vi "MainPanel_20170525.vi"() -> (0 "ErrorOut":errorcluster={"status"=TRUE, "code"=-63195, "source"="niLvFpga_Close_Dynamic.vi"})   [LabVIEW 2018]
doc: "This is the main application VI and is a good framework to begin all applications with. See block diagram for detailed documentation.\n\n\nCopyright © 2017 Epimedia, Inc. All Rights Reserved.\n\nThe Epimedia Application Library is Copyright © 2009-2017 Epimedia, Inc. \nAll Rights Reserved. Used under license."
uses:
  Controls/Clusts/FreqShift.ctl
  Controls/Enums/TargetNumber.ctl
  Controls/Clusts/ScaleTargetClust.ctl
  Controls/Clusts/FPGA_Scale.ctl
  Controls/RadioButtons/FilterEnableRadio.ctl
  Controls/Clusts/Inclinometer_User_Cfg.ctl
  Controls/Clusts/AlarmSettingsClust.ctl
  Controls/Clusts/AlarmThresh_OneChan.ctl
  Controls/Clusts/SaturationMonitor.ctl
  Queue/MainQueueElements.ctl
  Queue/HWQueueElements.ctl
  Queue/DataQueueElements.ctl
  Controls/MasterCluster.ctl
  Controls/Clusts/AdminCluster.ctl
  Controls/UserLevelEnum.ctl
  Controls/RT_Config.ctl
  Controls/SMSDataCluster.ctl
  Controls/Clusts/FPGA_Config_Clust.ctl
  Controls/Clusts/Config_Clust.ctl
  Controls/Clusts/UserConfig.ctl
  Controls/PathsCluster.ctl
  Controls/Clusts/FrontPanel_UserConfig.ctl
  Controls/Clusts/FP_UserTargetConfig.ctl
  Controls/Enums/ScaleMeasure.ctl
  Controls/SystemStatusCluster.ctl
  Controls/SystemStateEnum.ctl
  Controls/Enums/NoiseQueueElements.ctl
  Controls/Enums/DigiLoopEnum.ctl
  Controls/Enums/FP_Loop_Enum.ctl
  Controls/Enums/AI_Type_Enum.ctl
  Controls/Clusts/FP_Loop_Clust.ctl
  Controls/Clusts/DigOutClust.ctl
  Controls/Clusts/NoiseFLoorSums.ctl
  Controls/Clusts/PowerHistory_All.ctl
  Controls/Enums/10Hz_Loop_Enum.ctl
  Controls/Enums/TCP_Loop.ctl
  Controls/Enums/LogLoopEnum.ctl
  Controls/Clusts/HDF5_10HzRefs.ctl
  <vilib>/addons/h5labview2/base/hid_t.ctl
  Controls/Clusts/TargetToneData.ctl
  Controls/Clusts/ChannelToneData.ctl
  Controls/ToneInfoClust.ctl
  Controls/Enums/WatchdogTimer_Enum.ctl
  Controls/Clusts/NoiseFloorData.ctl
  Controls/Clusts/FPGA_Probes.ctl
  Controls/Clusts/PXI_Health.ctl
  Controls/Clusts/All_AI_Error_and_Data.ctl
  Controls/Clusts/AI_Clust.ctl
  Controls/Clusts/All_AI_Error_Status.ctl
  Controls/Clusts/ErrorStatus.ctl
  Controls/Clusts/All_TC_Error_and_Data.ctl
  HDF5/TC_Data_Structure.ctl
  Controls/Clusts/All_TC_Error_Status.ctl
  Controls/Clusts/AlarmDisplay.ctl
  Controls/Clusts/SerialMeasurements_Clust.ctl
  Controls/Clusts/Saturation_Status_Clust.ctl
  Controls/Enums/AI_Loop_Enum.ctl
  Controls/Enums/AO_Loop_Enum.ctl
  <vilib>/Utility/xml.llb/Write to XML File(string).vi
panel:
  out "TCP Connection":bool=TRUE
  out "Cx_Yell":bool
  out "Red":bool
  out "Rx_Yell":bool
  out "Green":bool=TRUE
  out "Logging to NAS":bool=TRUE
  out "10 MHzPLL Status":bool
  out "Input Over Range":bool=TRUE
  out "Auto Center":bool
  in  "Location":string caption="Connex Location"
  out "UTC date/time":string
  in  "Config":bool
  in  "SysErr":string="\nUnrecoverable System Error Handling Error!\n\nKey System File(s) are missing.\n"
  in  "RightSideTab":T1(tab)
  in  "AutoOffset":bool caption="Auto Offset"
  out "84 GHz":T2 {"MeasMax" format="%#.2g"; "MeasMean1" format="%#.2g"; "7_Max" format="%#.6g"; "6_Max" format="%#.2g"; "5_Max" format="%#.2g"; "4_Max" format="%#.2g"; "1_Max" format="%#.2g"; "MeasMean0" format="%#.2g"}
  in  "Scale":T3={"Measure"=0.050018310546875, "Step1"=2.0, "Scale"={"Step4"=3.0, "Step5"=1.0, "Step6"=1.0, "Step7"=1.0}} caption="Scale All Targets" {"Step1" format="%#_4g"; "Measure" format="%#_4g"}
  in  "FilterEnable":T5=enum."Step 1" caption="Enable Filter Stages"
  out "72 GHz":T2 {"MeasMax" format="%#.2g"; "MeasMean1" format="%#.2g"; "7_Max" format="%#.6g"; "6_Max" format="%#.2g"; "5_Max" format="%#.2g"; "4_Max" format="%#.2g"; "1_Max" format="%#.2g"; "MeasMean0" format="%#.2g"}
  out "Digitizer Offset 72 Co":fxp<+/-,16,16> caption="72 Co"
  out "Digitizer Offset 72 X":fxp<+/-,16,16> caption="72 X"
  out "Digitizer Offset 84 Co":fxp<+/-,16,16> caption="84 Co"
  out "Digitizer Offset 84 x":fxp<+/-,16,16> caption="84 x"
  in  "SimulateFPGA":bool caption="Simulate FPGA Signal"
  out "Voltages":string[][](table)=[["5V Aux", "4.50", "5.50", "4.99", "Yes"], ["3.3V Aux", "2.97", "3.63", "3.25", "Yes"], ["5V Backplane", "4.50", "5.50", "4.98", "Yes"], ["3.3V Backplane", "2.97", "3.63", "3.29", "Yes"], ["12V Backplane", "10.80", "13.20", "11.95", "Yes"], ["-12V Backplane", "-13.20", "-10.80", "-11.86", "Yes"], ["12V Fan", "10.80", "13.20", "12.01", "Yes"]]
  out "Fans":string[][](table)=[["Fan 1", "2438"], ["Fan 2", "2438"], ["Fan 3", "2443"], ["Fan 4", "2437"], ["Fan 5", "2436"], ["Fan 6", "2440"]]
  out "Temperatures":string[][](table)=[["Intake", "-20.00", "200.00", "32.00", "Yes"], ["Exhaust Temp1", "-40.00", "85.00", "51.23", "Yes"], ["Exhaust Temp2", "-40.00", "85.00", "40.30", "Yes"], ["Exhaust Temp3", "-40.00", "85.00", "37.18", "Yes"], ["Exhaust Temp4", "-40.00", "85.00", "40.30", "Yes"]]
  out "Combined Power History":T6(graph)
  in  "NewValueWeighting":dbl=0.75 min=0.01 max=1.0 step=0.01
  in  "Inclin":T7
  out "Inclinometer History":T8(graph)
  in  "LeftSideTab":T9(tab)
  in  "Deadband":dbl caption="Tracking Deadband (Hz)\nfull width" format="%#.0f"
  in  "MaxTrackRate":u32 caption="Track Rate (df/s)"
  in  "SNR_Thresh":dbl=-90.0 caption="Don't AutoCenter below this SNR level (dB)"
  in  "Tone Tabs":T10(tab)
  out "Cal":dbl[](graph)
  out "Beacon":dbl[][](graph)
  out "FreqShiftTab_72Co":enum32{"Auto", "Manual"}(tab)=enum."Manual"
  in  "Shift Cal":T11={"Fine"=-2000.0, "Coarse_"=25000000.0} {"Coarse_" format="%_9f"; "Fine" step=100.0 format="%^#_6g"}
  in  "Shift Beac":T11={"Fine"=0.0, "Coarse_"=25624000.0} {"Coarse_" format="%_9f"; "Fine" step=500.0 format="%^#_6g"}
  out "Channel Power Cal":dbl
  out "Channel Power Beac":dbl
  out "Peak Location Cal":dbl format="%^#_9g"
  out "Peak Location Beacon":dbl format="%^#_9g"
  out "SNR":dbl
  out "Beacon 2":dbl[](graph)
  out "Cal 2":dbl[](graph)
  out "Channel Power Beac 2":dbl
  out "Channel Power Cal 2":dbl
  out "Peak Location Cal 2":dbl format="%^#_9g"
  out "Peak Location Beacon 2":dbl format="%^#_9g"
  out "SNR 2":dbl
  out "Peak Location Cal 3":dbl format="%^#_9g"
  out "Peak Location Beacon 3":dbl format="%^#_9g"
  out "Channel Power Beac 3":dbl
  out "Channel Power Cal 3":dbl
  out "Cal 3":dbl[](graph)
  out "Beacon 3":dbl[][](graph)
  out "FreqShiftTab_84Co":enum32{"Auto", "Manual"}(tab)=enum."Manual"
  in  "Shift Cal 3":T11={"Fine"=-2000.0, "Coarse_"=25000000.0} {"Coarse_" format="%_9f"; "Fine" step=1000.0 format="%^#_6g"}
  in  "Shift Beac 3":T11={"Fine"=-1200.0, "Coarse_"=25508000.0} {"Coarse_" format="%_9f"; "Fine" step=3000.0 format="%^#_6g"}
  out "SNR 3":dbl
  out "Peak Location Cal 4":dbl=25000867.0 format="%^#_9g"
  out "Peak Location Beacon 4":dbl=26247708.0 format="%^#_9g"
  out "Channel Power Beac 4":dbl=-172.30831588057904
  out "Channel Power Cal 4":dbl=-172.65485177884602
  out "Cal 4":dbl[](graph)
  out "Beacon 4":dbl[](graph)
  out "SNR 4":dbl
  out "df (Hz)":dbl=1.0
  in  "Zoom On Peak":bool
  in  "AutoCenter":bool
  in  "AutoScale Y Tones":bool caption="AutoScale Y"
  out "Delta Phase 84 GHz":dbl(graph)
  out "Delta Phase 72 GHz":dbl(graph)
  out "84 X Beac":dbl(graph)
  out "84 Co Beac":dbl(graph)
  out "72 X Beac":dbl(graph)
  out "72 Co Beac":dbl(graph)
  in  "NoiseCalcTabs":enum32{"Sums", "Calculations"}(tab)
  out "Noise Floor Sum Histories":cluster{"1":dbl, "2":dbl, "3":dbl, "4":dbl}(graph)
  out "NoiseFloorSum 2":dbl=7.853169888502882e-06 caption="NoiseFloorSum 72 X" format="%^#.4g"
  out "NoiseFloorSum 4":dbl caption="NoiseFloorSum 84 X" format="%^#.4g"
  out "NoiseFloorSum 3":dbl=5.6412082576295616e-06 caption="NoiseFloorSum 84 Co" format="%^#.4g"
  out "NoiseFloorSum":dbl=1.7031731794048579e-06 caption="NoiseFloorSum 72 Co" format="%^#.4g"
  in  "FreqsToRemove 2":i32[](array[numeric])=[0, 1633] caption="Frequencies to remove [Hz]" format="%#.9f"
  in  "Width 2 [bins]":i32[](array[numeric])
  in  "FreqsToRemove":i32[](array[numeric])=[0, 1633] caption="Frequencies to remove [Hz]" format="%#.9f"
  in  "Width [bins]":i32[](array[numeric])
  in  "Noise Floor Tabs":T10(tab)=enum."84 GHz Cross"
  out "NoiseFloor":dbl[](graph)=[-66.50915074981145, -77.35517980815544, -70.92434771683105, -72.86535876954508, -107.5864217084241, -66.94671114313334, -86.9680791592285, -68.04380719104392, -71.14797089641604, -63.16968529661337, -82.48880594923583, -62.394262379750494, -69.41405540583582, -70.44999041078472, -62.764694502724275, -69.85852362169294, -61.20801118479691, -60.96232819890859, -67.0420916611973, -76.9325123260613, -71.20470080745599, -59.94612909219138, -67.09384592930908, -67.75357665166754, -63.68561668587035, -79.05247609152548, -64.30819977245869, -71.92525230951662, -62.60086763754057, -76.64734907877724, -67.28855831253992, -67.13098496137215, -59.47573928376156, -63.37374642804294, -58.85306181225433, -59.0113657345912, -64.58953958406045, -70.86924704839845, -79.26102778332853, -61.52216258278157, -80.3481898614786, -75.765935107876, -65.48046717202362, -69.19931261895289, -63.949032467233216, -63.75864694613728, -72.87889864476392, -56.79760525136199, -71.65909904633395, -59.06578970836555, -64.91475716928525, -57.19343570542245, -62.79306219219861, -55.81556426495866, -64.05645800193233, -65.73443303002963, -75.21456372039822, -86.01638976497799, -53.953967724982654, -62.330882253021905, -62.661391497611554, -55.735821494891475, -77.26914335701082, -83.54061295051198, -55.53376160252768, -59.37242649088039, -60.48906914982559, -75.0602494009469, -66.65904341140876, -77.75218818680568, -52.477623238047464, -66.00191924743532, -81.95073969565235, -55.208321856836896, -81.91591933074315, -73.83258325532779, -60.85727300175419, -75.67483280875109, -105.75362882215944, -63.135275318647835, -86.90940619345022, -56.06589110459543, -62.14321627753413, -65.89664521425757, -71.08033489355404, -88.42724907547671, -86.34160735020279, -68.07660380418503, -74.5954456871255, -60.31196258100402, -102.29042779841981, -58.54712285471978, -57.1066682233888, -63.68561668587035, -53.84157042278512, -64.07808822530168, -83.09809005033009, -67.86540306368099, -59.74416373775657, -57.42602087556475, -82.86505025051522, -83.4178863299571, -61.36992220129098, -63.283623635764734, -62.448923496303216, -64.15963873058894, -79.77530324298593, -76.62730100460487, -58.90659256005497, -57.12238586753852, -64.13237812685045, -70.84729509373918, -62.27688773899296, -66.60253072956394, -67.06423788111388, -57.29166293696944, -62.40335096403998, -81.985686910987, -80.43715185916025, -64.04566115217133, -92.88133277427832, -55.42331829191223, -55.120674896161084, -63.194339640689996, -61.59292923045107, -60.29735024002179, -53.54632146630568, -81.64181496888733, -61.82980546303049, -57.78161308733092, -73.11204950616451, -60.511439156076044, -60.66950707129386, -57.55954298568111, -72.55910236513691, -67.66661849545392, -73.15378851327321, -80.11491392918538, -76.8092600952713, -57.76758207707761, -59.68576391549755, -69.68214071607247, -58.27721758621551, -57.474854125813316, -57.792852690256986, -71.61149100817491, -57.59528138494674, -64.40853421412848, -59.10117046934344, -62.085865451395556, -64.29711600461678, -70.94647690772834, -59.96021573202071, -71.40013117318102, -91.0059778265747, -68.6782163581475, -85.80554611282477, -64.97400998274259, -62.950601935766436, -55.110040819027354, -59.39233587194578, -76.10125856709311, -70.38708526734541, -63.70121929164116, -61.167956846856164, -56.64922452409264, -63.135275318647835, -73.04288554397968, -75.91352263430315, -58.88136440613294, -95.07660997858827, -76.9325123260613, -55.1933009388814, -65.66391951508285, -53.42073336253301, -61.02513038720361, -79.20846326824847, -59.627717466812165, -78.74791082859372, -79.00103897097017, -56.92260555741537, -53.90697537079881, -122.53370302934468, -60.593911723440904, -59.84809758215223, -55.827010394463606, -70.85826479190422, -63.071696702033954, -67.59605258674068, -59.827220533651264, -76.40949391870066, -61.136033356497144, -93.32759928426387, -60.677099473747965, -64.04026728078941, -59.69261605864603, -66.99795201277061, -65.4491890223706, -81.985686910987, -62.33991095957074, -69.97794010149332, -66.42113041531445, -64.87938036213663, -60.47790367814803, -58.27721758621551, -61.95047372074091, -67.30370117282712, -55.47838100766122, -82.34234508908514, -64.4253591234399, -62.10347536914477, -64.12149553918309, -70.89124935162172, -64.06726701716042, -65.83143082306387, -71.28469055024624, -65.3374246513794, -83.54061295051198, -70.71662792027197, -79.02672305592466, -71.5169779283971, -66.49745848526379, -61.685291431907324, -90.91673997376512, -61.46839697534468, -55.97939338197404, -71.99913970945016, -70.59839337034478, -58.73757611624553, -69.25487068930309, -71.44669922579382, -86.62130646331073, -56.72690106185417, -64.79733832268226, -71.3307002307699, -80.55706592055753, -68.08482050704285, -61.989584533692884, -59.67891666324396, -68.02745083584529, -57.598036015259986, -76.85016847282978, -62.14321627753413, -88.29117587199889, -53.237129671891786, -53.739683783843354, -69.11657420476445, -63.92236300329483, -57.9116704876057, -85.85782417136002, -60.08079476870609, -63.434302126231735, -82.78861159907069, -67.65089226242378, -67.23574575288268, -54.48667245338559, -67.36451278692888, -60.70752931686879, -69.02547190563956, -61.79133938342206, -74.10582008083972, -62.34442850144843, -53.97471751185552, -51.333739549665786, -65.72800124970155, -85.10207921011511, -67.70604723982245, -81.91591933074315, -57.87190081264216, -72.98791118149637, -65.14189176731313, -63.11077211247754, -61.02513038720361, -77.3768100315248, -69.61441375800541, -57.31303415160058, -78.21347897550834, -59.99198650623064, -59.114068622547016, -62.61480082808004, -65.28816652004411, -67.22070969964764, -73.65465543441897, -71.34223721351944, -67.02735586720914, -73.65465543441897, -56.18403299187383, -57.523937234598, -67.25834411433442, -77.05736875236039, -62.398805595558834, -59.63452825872057, -69.50894243068942, -55.60288055349337, -80.20172900132795, -79.44730548095569, -55.63875065838558, -66.10836139358406, -58.72207603208485, -58.29497692482666, -59.08185569771779, -72.67778016739874, -65.52442862375423, -61.98087945142586, -58.25949106438673, -59.88998847841493, -60.749528587935266, -84.40154908991724, -66.44881586021592, -53.29676818907982, -52.73633391630178, -60.71896543982064, -53.09135769185345, -58.6265305032935, -73.75804519578128, -56.71935642914125, -68.61719752452004, -57.598036015259986, -53.3337898283395, -64.87349689062438, -88.29117587199889, -58.453295635683695, -57.28632756419565, -61.12011136114078, -78.28462639681322, -66.36599807965678, -76.64734907877724, -59.63452825872057, -66.75159255224662, -65.43670626198858, -64.71599198424335, -90.23123413228441, -71.70694453204936, -61.660013419915934, -74.24541348985224, -75.82101468502773, -55.70410906931722, -64.08350341031704, -68.94421306683006, -57.3264153784878, -68.89936492530401, -77.18387168443718, -60.79171254557675, -58.58369087867003, -67.73770733456635, -65.3497788063386, -62.12995100692533, -61.02119318214117, -66.23631485249587, -53.28621676730112, -69.5759262439922, -69.46138159950439, -62.394262379750494, -89.51441115362678, -59.01455861197133, -66.53934938152648, -59.398981525138474, -61.28457827894233, -63.179539432045864, -71.50522899857577, -53.402925672251335, -72.18638703360062, -65.8184409768001, -77.26914335701082, -77.618018167542, -74.4029375547791, -65.92285561307659, -59.696043966490244, -89.74745095344164, -59.57340451210353, -54.16158766254612, -66.37975148703052, -59.09794863891852, -70.30384830260698, -58.90659256005497, -60.522643751470916, -76.68757135992576, -63.298585427204195, -69.00735480865882, -67.54152462831524, -59.823745438521804, -59.2636574163325, -68.09304425379594, -65.96230597710542, -74.5630915249219, -62.03760420165235, -59.188571445108, -59.96021573202071, -62.23212330872112, -67.46416130580153, -75.72939030177491, -62.77414108152802, -66.8957425222851, -68.37693094025309, -100.44500423225278, -67.67449129031516, -49.330032478862485, -65.90974146202535, -63.84279660853401, -78.3084599494455, -88.84744763463866, -70.68423734363549, -71.03550770917977, -66.0350557225249, -61.77003579927264, -66.27027241007812, -53.80810643536217, -73.95306207593867, -86.73551019305384, -58.65109645781953, -75.16284930944386, -66.04169677505735, -68.53069558583377, -91.655027241384, -65.83143082306387, -73.09817676332747, -87.63833899908943, -57.84642138199265, -71.35378808788312, -68.462051285777, -66.56036362870307, -69.74057541452339, -64.89115814139384, -72.19900110510912, -89.82640613165822, -74.43475516272025, -74.35540814293401, -57.55131453628453, -55.07397287871715, -62.462637580125666, -65.03363105719274, -73.07049131842601, -56.80014006442999, -57.398998322484964, -64.85586809546422, -56.72690106185417, -63.92236300329483, -72.71766795875487, -69.27346178039309, -60.188461443220056, -61.325123563306455, -66.22953774165236, -56.500646437883866, -80.1437650787519, -61.8469511333678, -64.06726701716042, -67.21320050161253, -75.02629184336465, -69.9180460463688, -64.76239110734761, -63.949032467233216, -59.18206991995233, -69.8981641739671, -60.7380559933847, -75.63863276579386, -103.86658696945702, -75.58458755242262, -70.34537650598938, -67.16826833515842, -64.37497266386126, -59.97785317034083, -87.38915615802296, -80.77059142903238, -98.69599353792836, -58.90659256005497, -68.81916287895487, -62.085865451395556, -67.92989406287103, -59.526131625169576, -80.0574706437699, -135.8324248355678, -65.53702613048907, -88.29117587199889, -75.33632600787547, -60.239122443647425, -57.73678590295665, -69.06180907029892, -58.72517404599841, -65.9031911032867, -69.4994113817186, -66.88848334675899, -66.8957425222851, -80.67849792174991, -69.67243611231109, -67.92180893807722, -70.89124935162172, -56.272404337593876, -66.0350557225249, -67.48730486346835, -60.533861449104684, -71.40013117318102, -87.45084768896143, -62.93617275280035, -57.46669796831478, -67.73770733456635, -54.14619576193157, -59.322833066623296, -63.333587290377515, -67.62735114631548, -63.790116629908674, -82.60013795316792, -59.27677605085558, -87.26695068374008, -68.73962580425172, -73.07049131842601, -93.91631158685163, -65.54964020199756, -66.67322375397606, -69.95793383772494, -98.69599353792836, -64.62959392200116, -65.21475034538807, -62.48553804456986, -63.52074904041135, -62.07707260018416, -70.13951023655673, -101.45572765895832, -68.21725401669875, -68.06019148196103, -70.40800784924883, -60.377994964097574, -55.137713977017334, -100.68787796424607, -51.248087194935714, -107.5864217084241, -70.01807823536436, -58.629597809474696, -75.00935803490745, -58.405225381636875, -59.05937083893905, -57.0805292426387, -54.19244575107637, -68.99830907484383, -60.087935074208794, -70.02813906481302, -58.14797741957073, -77.75218818680568, -61.88133468272222, -75.19729458882193, -58.48346232720986, -67.96230287747952, -64.21988614528689, -91.09605360575071, -67.56485581127916, -70.18033157475108, -82.16235857104732, -79.36702886186643, -61.55123859551514, -70.01807823536436, -60.481624058260586, -61.16396059601728, -64.29157891932596, -58.73757611624553, -104.21546177998823, -74.69316809415548, -72.45482959936831, -66.00191924743532, -62.75525721716239, -57.57602108878802, -57.46669796831478, -55.027497121659216, -62.703517449668844, -81.64181496888733, -67.5182500515929, -75.80261966500962, -54.819036072233125, -64.75077027006947, -70.70581890504388, -83.49952937594134, -71.21608715894112, -64.38614680606821, -75.0602494009469, -60.246381619173555, -72.98791118149637, -75.40660471047872, -77.66253332862755, -79.00103897097017, -71.62337088585414, -60.57510560097021, -62.591590073954784, -61.064591569955944, -64.78567509936107, -68.15908926509849, -70.49215751164556, -62.81202069639284, -63.10098832784568, -62.19646155761465, -53.45465931692457, -58.48044138560088, -77.3120651288393, -64.59525140322293, -62.18756679573493, -66.82339677970347, -64.44221359336854, -69.45189766398155, -70.79263397718645, -52.913894075334916, -67.64303880312309, -62.62410087728153, -67.69025628975479, -66.57439874459362, -61.77003579927264, -69.04362328286206, -57.262355040266804, -66.82339677970347, -67.61168910202014, -98.30438814449556, -83.4178863299571, -83.17704522854666, -54.798436966186195, -58.85306181225433, -69.88823866868432, -54.344316996899984, -56.83061018004191, -73.53784424987055, -56.694250421615884, -77.3768100315248, -61.12011136114078, -66.78024978042882, -62.84052888973603, -56.629280649965246, -64.21988614528689, -67.91373062181037, -83.25665564394805, -57.43956075078359, -87.63833899908943, -72.24962391387751, -67.13843005293714, -65.82493370124425, -68.12600992197582, -68.3938946935684, -70.49215751164556, -72.98791118149637, -79.10419050247984, -61.45191415342013, -87.95920503059935, -85.34743785340319, -100.44500423225278, -80.64799551131347, -89.3621381151705, -78.33235286341585, -71.59962582422565, -80.73979525491143, -65.96230597710542, -65.92941941764332, -78.7980049372049, -66.16202866642189, -63.644133377982975, -53.93138266452109, -62.86435060547873, -68.25901725201172, -55.708633002435725, -59.16259174067152, -58.82484247502318, -82.71277721205894, -63.16968529661337, -62.02885545503593, -63.84279660853401, -55.688292083046385, -67.27343931807863, -71.97444728912444, -72.53292772406871, -82.41529601098756, -57.28899487965841, -57.10405111792992, -68.59983462385247, -58.0319784245468, -71.87630832579441, -83.91850426012235, -57.80410547747103, -63.37374642804294, -88.84744763463866, -59.918017716763366, -74.69316809415548, -55.84535265626591, -78.87364002021206, -86.23197187116676, -61.47664901886427, -63.84808055248474, -64.25290855311093, -56.84588160804815, -57.87190081264216, -59.83765337861649, -64.4534663805826, -58.072418713283206, -66.93212102625245, -61.8469511333678, -82.34234508908514, -71.3653528873549, -62.79306219219861, -63.00853668658856, -66.18223155209182, -76.74822277376467, -83.7487122170078, -84.44669270263915, -69.31075240072312, -58.47742139502029, -84.91021281439802, -56.42477335451931, -79.34041858128046, -60.341254206815755, -76.40949391870066, -57.68104489778134, -57.30501436570783, -59.319535936499754, -68.44496668642603, -65.65115437680541, -64.03487644052393, -64.76239110734761, -88.29117587199889, -60.79171254557675, -62.940980069362986, -70.08872663463373, -56.05415654655729, -77.9340514533578, -58.292014750957215, -90.39807312011936, -67.54929538613183, -72.86535876954508, -67.7774299586116, -61.28053315975948, -69.08002939866336, -76.17739388736501, -68.12600992197582, -68.20892314340054, -60.15963196998185, -59.027340759098955, -68.6345919082523, -93.55876709656178, -70.14969929752522, -78.89898481698907, -59.34925098349115, -76.00693135674362, -62.169801975843306, -52.934203892377774, -66.25667495918356, -59.91100272559154, -73.50886235471478, -79.00103897097017, -64.3973339793477, -89.43797250218225, -55.708633002435725, -129.1830639324562, -62.494713559377466, -72.3773621528131, -62.494713559377466, -86.67823838115231, -61.048787612510004, -65.35596185521524, -95.07660997858827, -96.88059503539597, -71.42338694214621, -118.64407624726303, -68.61719752452004, -58.72207603208485, -72.87889864476392, -103.52995593850753, -65.77311453405315, -59.13668220432704, -64.11062528306243, -61.345460649574996, -63.949032467233216, -70.49215751164556, -64.98590459059014, -60.677099473747965, -64.53260766621884, -86.23197187116676, -70.53451078132562, -69.19008414301271, -67.51050439109943, -63.409024114240346, -58.402228973678724, -60.52638152669841, -70.13951023655673, -58.82484247502318, -71.25032752842785, -73.12594233987437, -77.98006113388146, -71.70694453204936, -62.29934853127211, -61.81269038266543, -73.87758568344123, -57.350548724549206, -63.23887776557276, -71.25032752842785, -65.76665677547876, -66.47658143676281, -79.85908543492619, -64.1432730740749, -63.38884955370265, -82.9421028736071, -92.35119789774856, -72.19900110510912, -64.61240729453161, -55.96079327920069, -57.3264153784878, -61.31294197436795, -67.71395247306751, -65.61296056391032, -61.702180520776785, -60.64298088413722, -76.37041850825705, -66.73015567181764, -60.00968250829721, -63.26868514325725, -72.93325006494365, -69.08002939866336, -78.72296152974505, -60.86888914848134, -89.28689851378687, -72.50682430660166, -61.321061314674914, -96.24082467983021, -81.91591933074315, -78.04949207629258, -63.933021893280305, -58.19477263431451, -84.72210874836932, -64.1869770221034, -80.98897809597787, -61.136033356497144, -60.14165744720392, -69.22705143346099, -60.93108061427673, -66.65196109288848, -68.86363676482424, -74.66048322437624, -78.35630543516089, -63.68042145151646, -73.18171575279334, -61.76152759472378, -64.72757074243842, -79.18228862718027, -68.32621892788234, -73.95306207593867, -90.06724723306866, -73.07049131842601, -78.33235286341585, -68.31779292821895, -100.68787796424607, -66.38663559209809, -57.11452382639363, -60.56383959850097, -88.42724907547671, -59.86204089856047, -68.15908926509849, -66.12175009080275, -73.61068438722714, -73.72839138546041, -64.87349689062438, -72.27503584926745, -68.81029279048192, -61.685291431907324, -60.03806418580448, -78.7980049372049, -68.6345919082523, -53.46539775088171, -55.991036786729076, -62.183122505639226, -62.41244816718737, -63.02307520919954, -54.81697417002206, -71.7189432828319, -58.008946000517206, -83.33693226303731, -68.02745083584529, -89.90601654705961, -63.93835578276997, -72.3773621528131, -76.48812550649035, -58.65724778858496, -65.1661165276611, -65.87050623350748, -76.40949391870066, -68.462051285777, -80.70909762871608, -61.702180520776785, -79.52825954787548, -60.231868757101445, -74.90837815512327, -68.81029279048192, -75.69298418597361, -59.30635873662562, -70.59839337034478, -81.50764494962365, -77.2264127741092, -81.05229845789066, -71.19332795490877, -78.67325675533309, -60.639197409428355, -71.5405190445054, -57.900290889592746, -70.09886187065311, -90.39807312011936, -83.66493002506755, -67.89759436905697, -62.81202069639284, -70.35578670777062, -70.28315142294974, -69.06180907029892, -67.01999644989385, -73.49440417564034, -82.75061947020467, -62.18756679573493, -64.69865000904744, -75.60256881354482, -58.66956229605267, -84.53762229339509, -56.15791665350603, -75.51299766793579, -75.58458755242262, -105.75362882215944, -76.02572274375143, -87.38915615802296, -73.84756061980656, -65.2208469455297, -78.02629254866153, -78.5012905626727, -67.69025628975479, -73.43678838683073, -61.12408938317581, -76.89125204740046, -60.00968250829721, -60.49279386352023, -63.00369540462864, -84.3118942317391, -58.28017519376167, -72.2877671052834, -88.09061804452719, -80.2600452903387, -87.14628242602967, -77.75218818680568, -67.92989406287103, -69.52803298425346, -72.4289375458631, -122.53370302934468, -82.86505025051522, -80.43715185916025, -78.52566922890597, -64.01334332261618, -59.87949859218653, -62.994020164272435, -57.78723124268914, -56.94831717827518, -57.76758207707761, -56.05650231010976, -73.09817676332747, -91.655027241384, -70.49215751164556, -73.01535898276833, -55.46293156224214, -72.61166688021697, -62.75525721716239, -80.67849792174991, -76.44872914721853, -70.2213273636385, -67.44107344868831, -68.79257718064568, -71.68299196030429, -73.19570992011825, -69.30141614694483, -61.27244803496567, -76.70774592046345, -66.39352464086812, -62.35799390554727, -71.19332795490877, -65.58758224223078, -84.35661692346315, -60.81480040268996, -55.23197377961066, -94.67404741663125, -91.27878294010458, -60.65434026971557, -66.51140180167204, -76.87068826675005, -78.3084599494455, -74.46667865307927, -69.22705143346099, -72.78451840350414, -83.33693226303731, -59.40895864512259, -63.99185843121669, -66.58142401037813, -82.63753761067531, -70.59839337034478, -58.402228973678724, -57.773192018757946, -68.32621892788234, -64.30819977245869, -77.84268885802032, -64.21439344545175, -61.989584533692884, -64.25290855311093, -83.05885482181219, -61.963492949158585, -56.272404337593876, -61.98523100514074, 
